vi "second_fp.vi"(0 "Waveform chart data":T1, 3 "Stat of sensors":T3) -> ()   [LabVIEW 2016]
panel:
  in  "Tab Control":enum32{"Page 1"}(tab)
  out "Waveform Chart":T1(graph)
  out "Status of sensors":T2
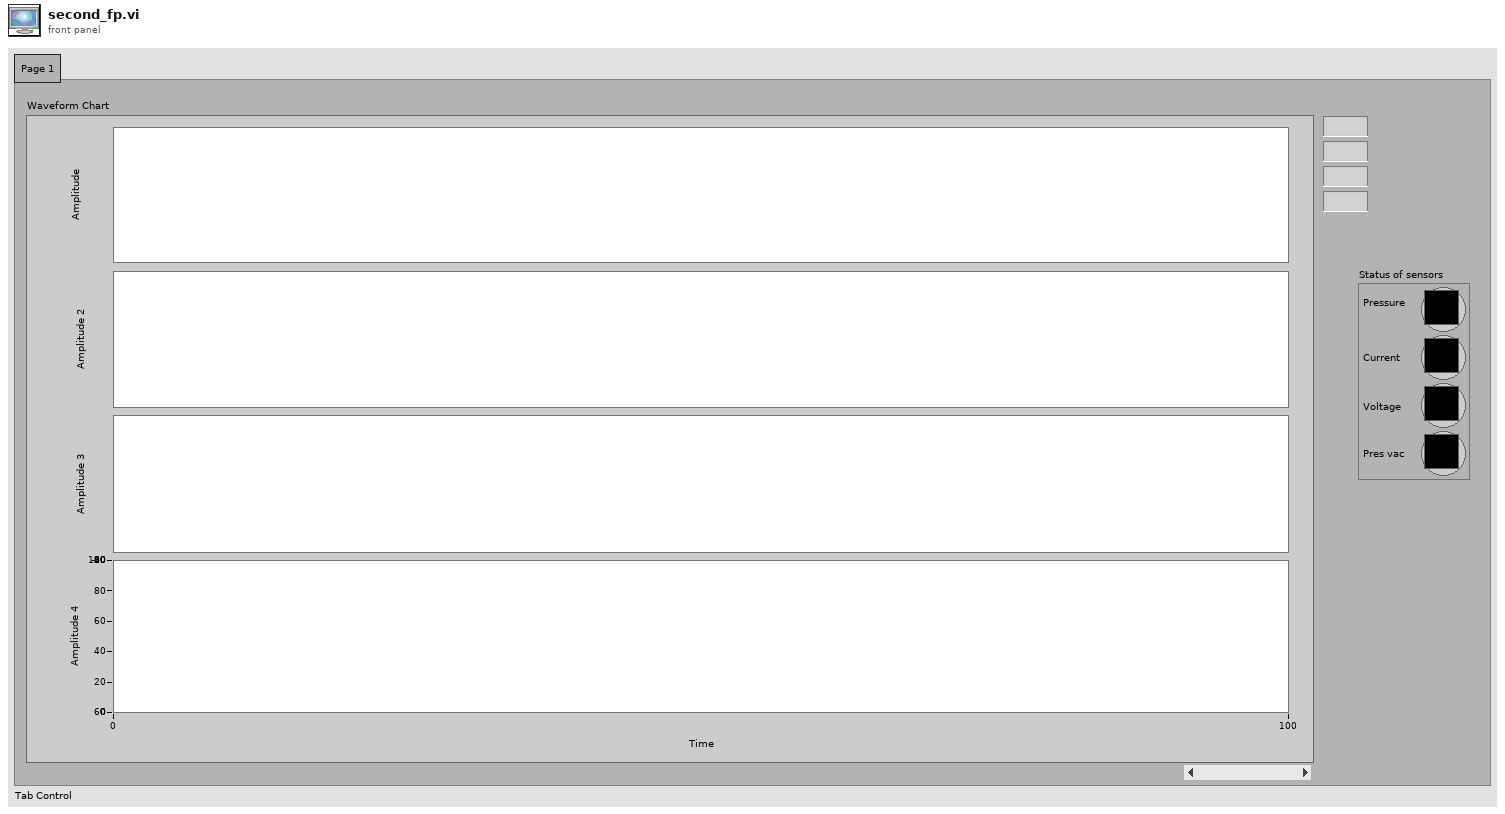
[diagram p1: front panel]
types:
  T1 = cluster{"[0]":dbl, "[1]":dbl, "[2]":dbl, "[3]":dbl}
  T2 = cluster{"Pressure":u32, "Current":u32, "Voltage":u32, "Pres vac":u32}
  T3 = cluster{"[0]":u32, "[1]":u32, "[2]":u32, "[3]":u32}
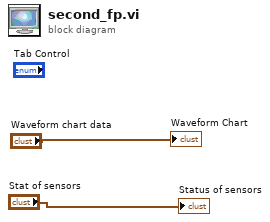
[diagram p0: block diagram]
diagram:
  "Waveform Chart" <- "Waveform chart data"
  "Status of sensors" <- "Stat of sensors"
